vi "TURCK GUI TestPanel IO-Link.vi"() -> ()   [LabVIEW 2017]
doc: "example for writing values to the TBEN-S2-4AO modul from Turck"
uses:
  KH TURCK ETHERNETIP TDef Enum IOL Data.ctl
  KH EthernetIP 17.19/KH_EthernetIP_Globals.vi
panel:
  out "error out":errorcluster
  in  "Output_IOL":T1={"IOL Port 1"=[0, 1], "IOL Port 3"=[0, 1], "IOL Port 5"=[0, 1], "IOL Port 7"=[0, 1]}
  out "Data_IOL":T2
  in  "DXP":bool[](array[boolean])=[FALSE, FALSE, FALSE, FALSE]
  in  "Exit":bool
  # "- Before starting the VI your PC has to be in the same subnet as the modules"
  # "Kirschenhofer Maschinen GmbH\nRömerstraße 35, 89278 Nersingen-Straß\ninfo@kirschenhofer-gmbh.de"
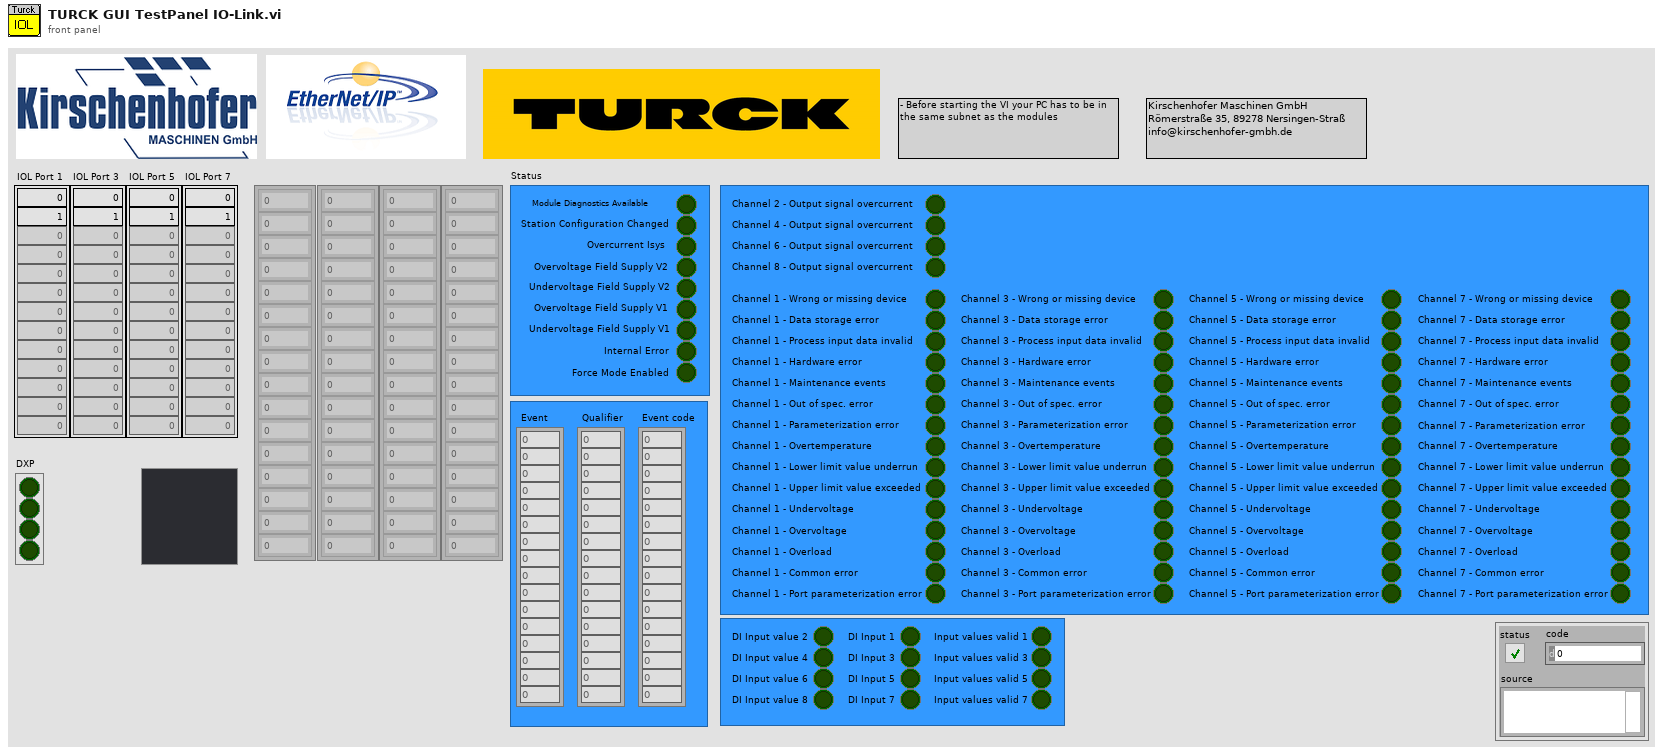
[diagram p1: front panel]
types:
  T1 = cluster{"IOL Port 1":u16[], "IOL Port 3":u16[], "IOL Port 5":u16[], "IOL Port 7":u16[]}
  T2 = typedef "KH TURCK ETHERNETIP TDef Enum IOL Data.ctl" = cluster{"Data_Port1":u16[], "Data_Port3":u16[], "Data_Port5":u16[], "Data_Port7":u16[], "Status":cluster{"Undervoltage Field Supply V2":bool, "Overvoltage Field Supply V1":bool, "Undervoltage Field Supply V1":bool, "Internal Error":bool, "Module Diagnostics Available":bool, "Station Configuration Changed":bool, "Overcurrent Isys":bool, "Overvoltage Field Supply V2":bool, "Force Mode Enabled":bool}, "Diagnostics":cluster{"Channel 2 - Output signal overcurrent":bool, "Channel 4 - Output signal overcurrent":bool, "Channel 6 - Output signal overcurrent":bool, "Channel 8 - Output signal overcurrent":bool, "Channel 1 - Wrong or missing device":bool, "Channel 3 - Wrong or missing device":bool, "Channel 5 - Wrong or missing device":bool, "Channel 7 - Wrong or missing device":bool, "Channel 1 - Data storage error":bool, "Channel 3 - Data storage error":bool, "Channel 5 - Data storage error":bool, "Channel 7 - Data storage error":bool, "Channel 1 - Process input data invalid":bool, "Channel 3 - Process input data invalid":bool, "Channel 5 - Process input data invalid":bool, "Channel 7 - Process input data invalid":bool, "Channel 1 - Hardware error":bool, "Channel 3 - Hardware error":bool, "Channel 5 - Hardware error":bool, "Channel 7 - Hardware error":bool, "Channel 1 - Maintenance events":bool, "Channel 3 - Maintenance events":bool, "Channel 5 - Maintenance events":bool, "Channel 7 - Maintenance events":bool, "Channel 1 - Out of spec. error":bool, "Channel 3 - Out of spec. error":bool, "Channel 5 - Out of spec. error":bool, "Channel 7 - Out of spec. error":bool, "Channel 1 - Parameterization error":bool, "Channel 3 - Parameterization error":bool, "Channel 5 - Parameterization error":bool, "Channel 1 - Overtemperature":bool, "Channel 3 - Overtemperature":bool, "Channel 5 - Overtemperature":bool, "Channel 7 - Overtemperature":bool, "Channel 1 - Lower limit value underrun":bool, "Channel 3 - Lower limit value underrun":bool, "Channel 5 - Lower limit value underrun":bool, "Channel 7 - Lower limit value underrun":bool, "Channel 1 - Upper limit value exceeded":bool, "Channel 3 - Upper limit value exceeded":bool, "Channel 5 - Upper limit value exceeded":bool, "Channel 7 - Upper limit value exceeded":bool, "Channel 1 - Undervoltage":bool, "Channel 3 - Undervoltage":bool, "Channel 5 - Undervoltage":bool, "Channel 7 - Undervoltage":bool, "Channel 1 - Overvoltage":bool, "Channel 3 - Overvoltage":bool, "Channel 5 - Overvoltage":bool, "Channel 7 - Overvoltage":bool, "Channel 1 - Overload":bool, "Channel 3 - Overload":bool, "Channel 5 - Overload":bool, "Channel 7 - Overload":bool, "Channel 1 - Common error":bool, "Channel 3 - Common error":bool, "Channel 5 - Common error":bool, "Channel 7 - Common error":bool, "Channel 1 - Port parameterization error":bool, "Channel 3 - Port parameterization error":bool, "Channel 5 - Port parameterization error":bool, "Channel 7 - Parameterization error":bool, "Channel 7 - Port parameterization error":bool}, "Events":cluster{"Event":u8[], "Qualifier":u8[], " Event code":u16[]}, "DXP":cluster{"DI Input value 2":bool, "DI Input value 4":bool, "DI Input value 6":bool, "DI Input value 8":bool, "DI Input 1":bool, "DI Input 3":bool, "DI Input 5":bool, "DI Input 7":bool, "Input values valid 1":bool, "Input values valid 3":bool, "Input values valid 5":bool, "Input values valid 7":bool}}
  T3 = cluster{"ItemCount":u16, "AdressItem":cluster{"TypeID":u16, "Length":u16, "Data":cluster{"ConnectionIdentifier":u32, "SequenceNumber":u32}}, "DataItem":cluster{"TypeID":u16, "Length":u16, "Data":u8[], "Sequence Count":u16}}
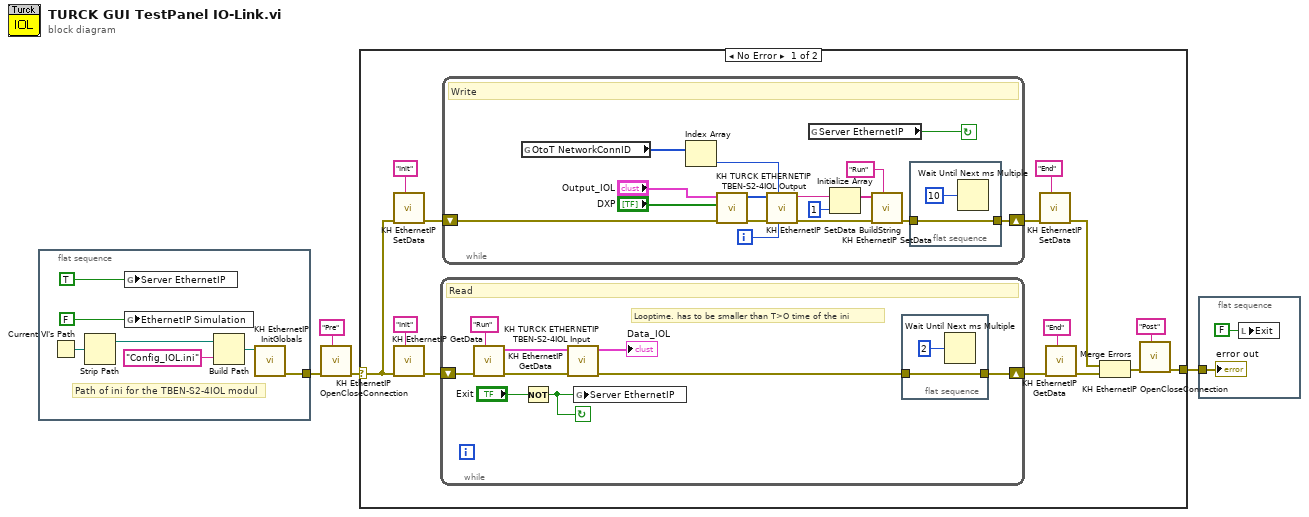
[diagram p0: block diagram]
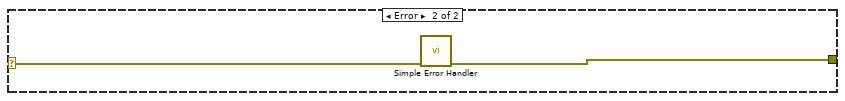
[diagram p2: hidden frame]
diagram:
  n1 = flat-sequence {
    tunnel: [w11] -> w2
    frame #0 {
      # "Path of ini for the TBEN-S2-4IOL modul"
      n2 = Current VI's Path() -> (path=w7:path)
      n3 = Strip Path(path=w7) -> (stripped path=w9:path)  [unwired: 1 out]
      n4 = global write "KH_EthernetIP_Globals.vi" "Server EthernetIP"(TRUE ("Server EthernetIP")) -> ()
      n5 = global write "KH_EthernetIP_Globals.vi" "EthernetIP Simulation"(FALSE ("EthernetIP Simulation")) -> ()
      n6 = Build Path(base path=w9, name or relative path="Config_IOL.ini") -> (appended path=w5:path)
      n7 = call "KH EthernetIP InitGlobals.vi"("Config File"=w5) -> ("err out"=w11:errorcluster)  [unwired: 10 in]
    }
  }
  n8 = call "KH EthernetIP OpenCloseConnection.vi"("Function"="Pre", "error in"=w2) -> ("error out"=w1:errorcluster)  [unwired: 9 in]
  n9 = case shown="No Error" w1 {
    selector: w1 -> [w12 w56]
    tunnel: [w13 w55] -> w3
    frame No Error {
      n10 = call "KH EthernetIP SetData.vi"("Function"="Init", "error in"=w12) -> ("error out"=w24:errorcluster)  [unwired: 7 in, 2 out]
      n11 = call "KH EthernetIP GetData.vi"("Function"="Init", "error in"=w12) -> ("error out"=w14:errorcluster)  [unwired: 8 in, 1 out]
      n12 = while {
        shift-right: [w50] -> w16
        shift-left: w14 -> [w52]
        stop <- w48 continue-if-true
        # "Looptime. has to be smaller than T>O time of the ini"
        # "Read"
        n13 = call "KH EthernetIP GetData.vi"("Function"="Run", "error in"=w52) -> ("error out"=w47:errorcluster, "Response Data"=w45:T3)  [unwired: 8 in]
        n14 = Not(x="Exit") -> (.not. x?=w48:bool)
        n15 = call "KH TURCK ETHERNETIP TBEN-S2-4IOL Input.vi"("error in"=w47, "Response Data"=w45) -> ("error out"=w46:errorcluster, "Data_IOL"=→"Data_IOL":T2)  [unwired: 8 in]
        n16 = global write "KH_EthernetIP_Globals.vi" "Server EthernetIP"(w48) -> ()
        n17 = flat-sequence {
          tunnel: w46 -> [w53]
          tunnel: [w53] -> w50
          frame #0 {
            n18 = Wait Until Next ms Multiple(millisecond multiple=u32 2) -> ()  [unwired: 1 out]
          }
        }
      }
      n19 = while {
        shift-right: [w41] -> w23
        shift-left: w24 -> [w38]
        i -> [w39]
        stop <- w40 continue-if-true
        # "Write"
        n20 = global read "KH_EthernetIP_Globals.vi" "OtoT NetworkConnID"() -> (w26:u32[])
        n21 = Index Array(array=w26) -> (element=w27:u32)  [unwired: 1 in]
        n22 = call "KH TURCK ETHERNETIP TBEN-S2-4IOL Output.vi"("error in"=w38, "DXP"="DXP", "Output_IOL"="Output_IOL") -> ("error out"=w31:errorcluster, "Output Data"=w30:u8[])  [unwired: 7 in]
        n23 = call "KH EthernetIP SetData BuildString.vi"("LoopIndex"=w39, "OtoT NetworkConnID"=w27, "error in"=w31, "Output Data"=w30) -> ("error out"=w32:errorcluster, "DataString"=w35:string)  [unwired: 6 in]
        n24 = global read "KH_EthernetIP_Globals.vi" "Server EthernetIP"() -> (w40:bool)
        n25 = Initialize Array(w35, 1 ("dimension size")) -> (w33:string[])
        n26 = call "KH EthernetIP SetData.vi"("Function"="Run", "error in"=w32, "Data Strings"=w33) -> ("error out"=w36:errorcluster)  [unwired: 6 in, 2 out]
        n27 = flat-sequence {
          tunnel: w36 -> [w42]
          tunnel: [w42] -> w41
          frame #0 {
            n28 = Wait Until Next ms Multiple(millisecond multiple=u32 10) -> ()  [unwired: 1 out]
          }
        }
      }
      n29 = call "KH EthernetIP SetData.vi"("Function"="End", "error in"=w23) -> ("error out"=w19:errorcluster)  [unwired: 7 in, 2 out]
      n30 = call "KH EthernetIP GetData.vi"("Function"="End", "error in"=w16) -> ("error out"=w21:errorcluster)  [unwired: 8 in, 1 out]
      n31 = Merge Errors(w19, w21) -> (w20:errorcluster)
      n32 = call "KH EthernetIP OpenCloseConnection.vi"("Function"="Post", "error in"=w20) -> ("error out"=w13:errorcluster)  [unwired: 9 in]
    }
    frame Error {
      n33 = call <vilib>:"Simple Error Handler.vi"("error in (no error)"=w56) -> ("error out"=w55:errorcluster)  [unwired: 4 in, 4 out]
    }
  }
  n34 = flat-sequence {
    tunnel: w3 -> [w57]
    frame #0 {
      n35 = local write "Exit"(FALSE ("Exit")) -> ()
      "error out" <- w57
    }
  }
